vi "setSerializedData.vi"(0 "reference":refnum<class "ClassRelationshipEdge.lvclass">, 1 "startNode":refnum<class "AbstractNode.lvclass">, 2 "endNode":refnum<class "AbstractNode.lvclass">, 3 "xmlOut":string, 5 "error in (no error)":errorcluster) -> (14 "reference out":refnum<class "ClassRelationshipEdge.lvclass">, 19 "error out":errorcluster)   [LabVIEW 2020, in "ClassRelationshipEdge.lvclass"]
uses:
  <resource>/Framework/Providers/Open_GDS/UML/ClassRelationshipEdge_class/ClassRelationshipEdge.lvclass
  C:/Program Files (x86)/National Instruments/LabVIEW 2020/resource/Framework/Providers/Open_GDS/UML/SegmentedLineEdge_class/SegmentedLineEdge.lvclass
  C:/Program Files (x86)/National Instruments/LabVIEW 2020/resource/Framework/Providers/Open_GDS/UML/AbstractEdge_class/AbstractEdge.lvclass
  <resource>/Framework/Providers/Open_GDS/UML/AbstractNode_class/AbstractNode.lvclass
  <resource>/Framework/Providers/Open_GDS/UML/General/Point/Point Point2D.ctl
  <resource>/Framework/Providers/Open_GDS/UML/LineStyle_class/LineStyleType.ctl
  <resource>/Framework/Providers/Open_GDS/UML/ArrowHead_class/ArrowHeadType.ctl
  <resource>/Framework/Providers/Open_GDS/UML/BentStyle_class/BentStyleType.ctl
  <resource>/Framework/Providers/Open_GDS/UML/LineStyle_class/LineStyle.lvclass
  <resource>/Framework/Providers/Open_GDS/UML/ArrowHead_class/ArrowHead.lvclass
  <resource>/Framework/Providers/Open_GDS/UML/BentStyle_class/BentStyle.lvclass
  <resource>/Framework/Providers/Open_GDS/UML/SegmentedLineEdge_class/SegmentedLineEdge.lvclass
  <resource>/Framework/Providers/Open_GDS/UML/AbstractEdge_class/AbstractEdge.lvclass
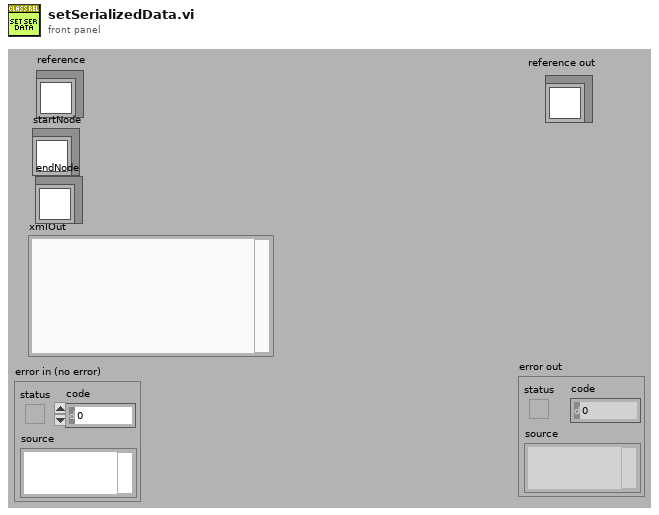
[diagram p1: front panel]
types:
  T1 = typedef "Point Point2D.ctl" = cluster{"x":dbl, "y":dbl}
  T2 = cluster{"Base class":cluster{"Base class":cluster{"Base class":cluster{"start":refnum<k1>, "end":refnum<k1>}}, "lineStyle":refnum<k1>, "startArrowHead":refnum<k1>, "endArrowHead":refnum<k1>, "startLabel":string, "midLabel":string, "endLabel":string, "MidLabelOffset":T1, "SplitWire":bool}, "bentStyleRef":refnum<k1>, "startConnectionOffset":cluster{"x":i32, "y":i32}, "endConnectionOffset":cluster{"x":i32, "y":i32}, "MidLineOffset":cluster{"x":i32, "y":i32}, "DepClass":cluster{"ThisVIs/Ctls":path[], "Dependent_VIs/Ctls":path[]}}
  T3 = typedef "ArrowHead.lvclass/ArrowHeadType.ctl" = enum16{"NONE", "TRIANGLE", "BLACK_TRIANGLE", "V", "HALF_V", "DIAMOND", "BLACK_DIAMOND"}
  T4 = typedef "BentStyle.lvclass/BentStyleType.ctl" = enum16{"STRAIGHT", "HV", "VH", "HVH", "VHV", "ARC"}
  T5 = typedef "LineStyle.lvclass/LineStyleType.ctl" = enum16{"SOLID", "DOTTED"}
  T6 = cluster{"Attributes":cluster{"Base class":cluster{"Base class":cluster{"Base class":cluster{"start":refnum<k1>, "end":refnum<k1>}}, "lineStyle":refnum<k1>, "startArrowHead":refnum<k1>, "endArrowHead":refnum<k1>, "startLabel":string, "midLabel":string, "endLabel":string, "MidLabelOffset":T1, "SplitWire":bool}, "bentStyleRef":refnum<k1>, "startConnectionOffset":cluster{"x":i32, "y":i32}, "endConnectionOffset":cluster{"x":i32, "y":i32}, "MidLineOffset":cluster{"x":i32, "y":i32}, "DepClass":cluster{"ThisVIs/Ctls":path[], "Dependent_VIs/Ctls":path[]}}, string, string, string, string}
  T7 = typedef "ClassRelationshipEdge.lvclass/ObjectAttributes.ctl" = cluster{"bentStyleRef":refnum<class "BentStyle.lvclass">, "startConnectionOffset":cluster{"x":i32, "y":i32}, "endConnectionOffset":cluster{"x":i32, "y":i32}, "MidLineOffset":cluster{"x":i32, "y":i32}, "DepClass":T8}
  T8 = typedef "ReversedEngineering_ViDependencyDetailsType.ctl" = cluster{"ThisVIs/Ctls":path[], "Dependent_VIs/Ctls":path[]}
  T9 = typedef "SegmentedLineEdge.lvclass/ObjectAttributes.ctl" = cluster{"lineStyle":refnum<class "LineStyle.lvclass">, "startArrowHead":refnum<class "ArrowHead.lvclass">, "endArrowHead":refnum<class "ArrowHead.lvclass">, "startLabel":string, "midLabel":string, "endLabel":string, "MidLabelOffset":T1, "SplitWire":bool}
  T10 = typedef "AbstractEdge.lvclass/ObjectAttributes.ctl" = cluster{"start":refnum<class "AbstractNode.lvclass">, "end":refnum<class "AbstractNode.lvclass">}
  T11 = cluster{"ThisVIs/Ctls":path[], "Dependent_VIs/Ctls":path[]}
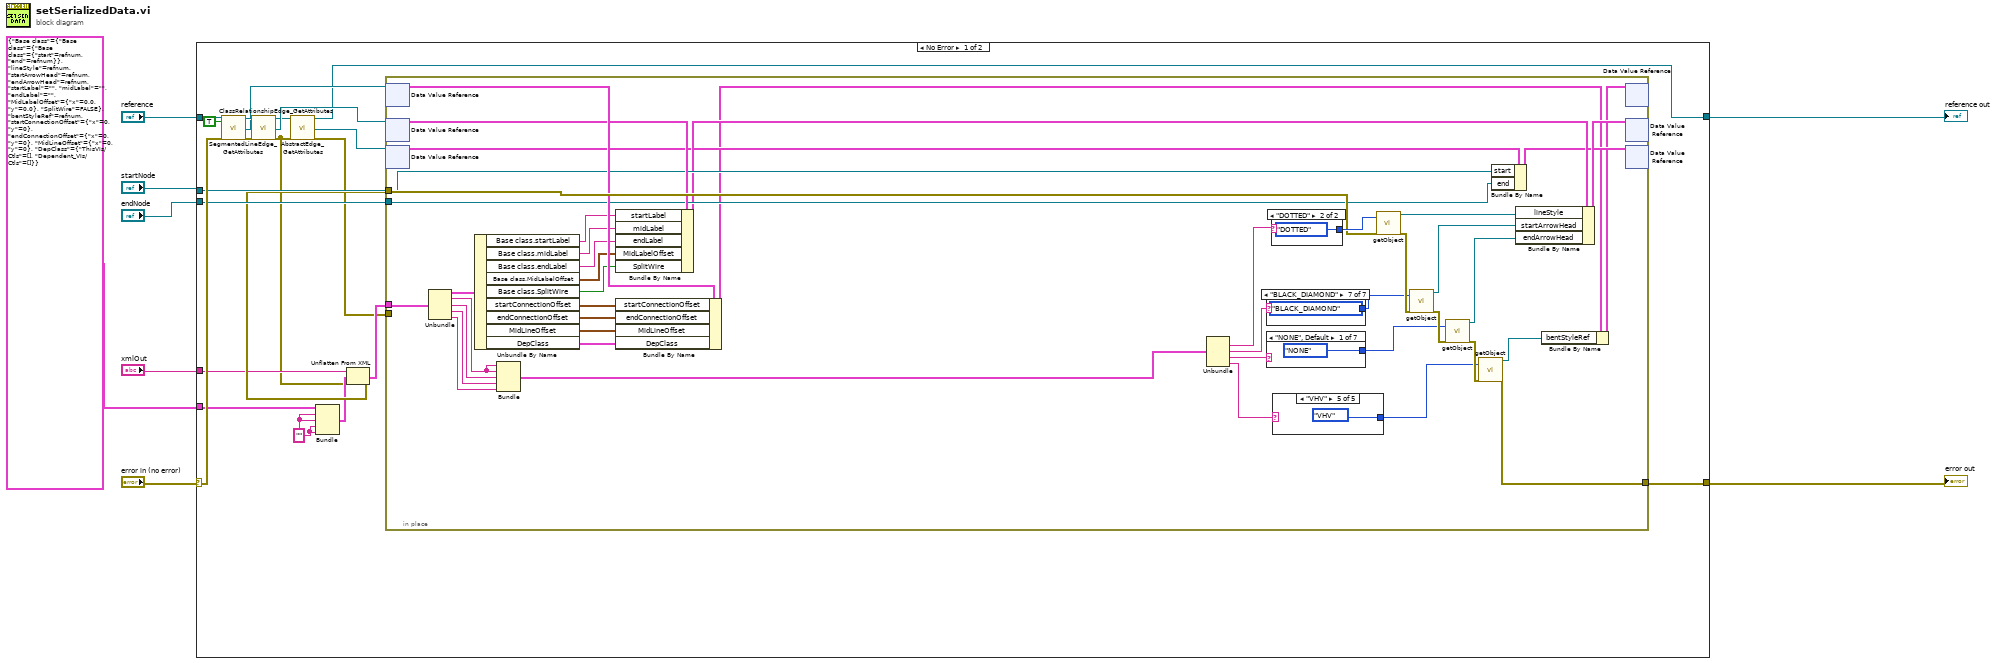
[diagram p0: block diagram]
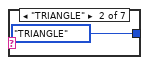
[diagram p2: hidden frame]
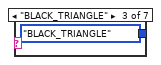
[diagram p3: hidden frame]
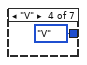
[diagram p4: hidden frame]
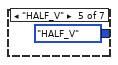
[diagram p5: hidden frame]
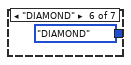
[diagram p6: hidden frame]
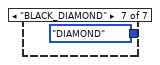
[diagram p7: hidden frame]
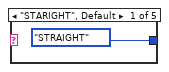
[diagram p8: hidden frame]
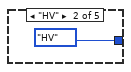
[diagram p9: hidden frame]
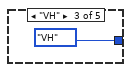
[diagram p10: hidden frame]
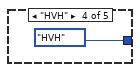
[diagram p11: hidden frame]
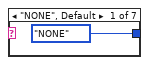
[diagram p12: hidden frame]
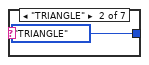
[diagram p13: hidden frame]
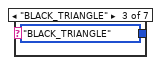
[diagram p14: hidden frame]
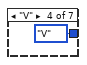
[diagram p15: hidden frame]
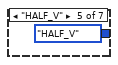
[diagram p16: hidden frame]
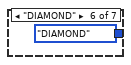
[diagram p17: hidden frame]
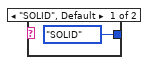
[diagram p18: hidden frame]
diagram:
  n1 = case shown="No Error" "error in (no error)" {
    selector: "error in (no error)" -> [w28 w94]
    tunnel: "reference" -> [w29 w95]
    tunnel: [w9 w95] -> w6
    tunnel: [w16 w94] -> w5
    tunnel: "xmlOut" -> [w18 _]
    tunnel: "startNode" -> [w27 _]
    tunnel: "endNode" -> [w26 _]
    tunnel: T2 {"Base class"={"Base class"={"Base class"={"start"=refnum, "end"=refnum}}, "lineStyle"=refnum, "startArrowHead"=refnum, "endArrowHead"=refnum, "startLabel"="", "midLabel"="", "endLabel"="", "MidLabelOffset"={"x"=0.0, "y"=0.0}, "SplitWire"=FALSE}, "bentStyleRef"=refnum, "startConnectionOffset"={"x"=0, "y"=0}, "endConnectionOffset"={"x"=0, "y"=0}, "MidLineOffset"={"x"=0, "y"=0}, "DepClass"={"ThisVIs/Ctls"=[], "Dependent_VIs/Ctls"=[]}} ("Attributes") -> [w24 _]
    frame No Error {
      w25 = ""
      n2 = call <resource>:"ClassRelationshipEdge_GetAttributes.vi"("reference in"=w29, "OnlyGetDvrReference(False)"=TRUE, "error in (no error)"=w28) -> ("reference out"=w22:refnum<class "ClassRelationshipEdge.lvclass">, "DataRef"=w13:refnum<data-value>, "error out"=w21:errorcluster)  [unwired: 13 in, 1 out]
      n3 = call <resource>:"SegmentedLineEdge_GetAttributes.vi"("reference in"=w22, "error in (no error)"=w21) -> ("reference out"=w10:refnum<class "ClassRelationshipEdge.lvclass">, "DataRef"=w12:refnum<data-value>, "error out"=w15:errorcluster)  [unwired: 14 in, 1 out]
      n4 = call <resource>:"AbstractEdge_GetAttributes.vi"("reference in"=w10, "error in (no error)"=w15) -> ("reference out"=w9:refnum<class "ClassRelationshipEdge.lvclass">, "DataRef"=w11:refnum<data-value>, "error out"=w14:errorcluster)  [unwired: 14 in, 1 out]
      n5 = Bundle("Attributes"=w24, w25, w25, w25, w25) -> (w17:T6)  [unwired: 1 out]
      n6 = Unflatten From XML(xml string=w18, type=w17, error in (no error)=w15) -> (value=w19:T6, error out=w20:errorcluster)
      n7 = in-place {
        in-place-border: w27 -> [w53]
        in-place-border: w26 -> [w52]
        in-place-border: w20 -> [w57]
        in-place-border: w19 -> [w58]
        in-place-border: w14 -> [_]
        in-place-border: [w56] -> w16
        n8 = in-place-dvr #1(w13) -> (w55:T7)  [unwired: 1 out]
        n9 = in-place-dvr #2(w12) -> (w54:T9)  [unwired: 1 out]
        n10 = in-place-dvr #3(w11) -> (w49:T10)  [unwired: 1 out]
        n11 = Unbundle(w58) -> ("Attributes"=w41:T2, w31:string, w42:string, w43:string, w44:string)
        n12 = Unbundle By Name(w41) -> ("Base class.startLabel"=w40:string, "Base class.midLabel"=w39:string, "Base class.endLabel"=w38:string, "Base class.MidLabelOffset"=w37:T1, "Base class.SplitWire"=w36:bool, "startConnectionOffset"=w35:cluster{"x":i32, "y":i32}, "endConnectionOffset"=w34:cluster{"x":i32, "y":i32}, "MidLineOffset"=w33:cluster{"x":i32, "y":i32}, "DepClass"=w32:T11)
        n13 = Bundle(w31, w31, w42, w43, w44) -> (w30:cluster{string, string, string, string, string})  [unwired: 1 out]
        n14 = Bundle By Name(cluster=w54, "startLabel"=w40, "midLabel"=w39, "endLabel"=w38, "MidLabelOffset"=w37, "SplitWire"=w36) -> (w50:T9)
        n15 = Bundle By Name(cluster=w55, "startConnectionOffset"=w35, "endConnectionOffset"=w34, "MidLineOffset"=w33, "DepClass"=w32) -> (w46:T7)
        n16 = Unbundle(w30) -> (w66:string, w62:string, w60:string, w61:string)  [unwired: 1 out]
        n17 = case shown="\"BLACK_DIAMOND\"" w62 {
          tunnel: [ArrowHeadType."NONE" ("arrowHead") ArrowHeadType."TRIANGLE" ("arrowHead") ArrowHeadType."BLACK_TRIANGLE" ("arrowHead") ArrowHeadType."V" ("arrowHead") ArrowHeadType."HALF_V" ("arrowHead") ArrowHeadType."DIAMOND" ("arrowHead") ArrowHeadType."BLACK_DIAMOND" ("arrowHead")] -> w64
          frame "NONE", Default {
          }
          frame "TRIANGLE" {
          }
          frame "BLACK_TRIANGLE" {
          }
          frame "V" {
          }
          frame "HALF_V" {
          }
          frame "DIAMOND" {
          }
          frame "BLACK_DIAMOND" {
          }
        }
        n18 = case shown="\"NONE\", Default" w60 {
          tunnel: [ArrowHeadType."NONE" ("arrowHead") ArrowHeadType."TRIANGLE" ("arrowHead") ArrowHeadType."BLACK_TRIANGLE" ("arrowHead") ArrowHeadType."V" ("arrowHead") ArrowHeadType."HALF_V" ("arrowHead") ArrowHeadType."DIAMOND" ("arrowHead") ArrowHeadType."DIAMOND" ("arrowHead")] -> w59
          frame "NONE", Default {
          }
          frame "TRIANGLE" {
          }
          frame "BLACK_TRIANGLE" {
          }
          frame "V" {
          }
          frame "HALF_V" {
          }
          frame "DIAMOND" {
          }
          frame "BLACK_DIAMOND" {
          }
        }
        n19 = case shown="\"DOTTED\"" w66 {
          tunnel: [LineStyleType."SOLID" ("lineStyle") LineStyleType."DOTTED" ("lineStyle")] -> w65
          frame "SOLID", Default {
          }
          frame "DOTTED" {
          }
        }
        n20 = case shown="\"VHV\"" w61 {
          tunnel: [BentStyleType."STRAIGHT" ("bentStyle") BentStyleType."HV" ("bentStyle") BentStyleType."VH" ("bentStyle") BentStyleType."HVH" ("bentStyle") BentStyleType."VHV" ("bentStyle")] -> w63
          frame "STARIGHT", Default {
          }
          frame "HV" {
          }
          frame "VH" {
          }
          frame "HVH" {
          }
          frame "VHV" {
          }
        }
        n21 = call <resource>:"getObject.vi"("lineStyle"=w65, "error in (no error)"=w57) -> ("reference out"=w72:refnum<class "LineStyle.lvclass">, "error out"=w71:errorcluster)  [unwired: 16 out]
        n22 = call <resource>:"getObject.vi"("arrowHead"=w64, "error in (no error)"=w71) -> ("reference out"=w68:refnum<class "ArrowHead.lvclass">, "error out"=w70:errorcluster)  [unwired: 16 out]
        n23 = call <resource>:"getObject.vi"("arrowHead"=w59, "error in (no error)"=w70) -> ("reference out"=w69:refnum<class "ArrowHead.lvclass">, "error out"=w67:errorcluster)  [unwired: 16 out]
        n24 = call <resource>:"getObject.vi"("bentStyle"=w63, "error in (no error)"=w67) -> ("reference out"=w45:refnum<class "BentStyle.lvclass">, "error out"=w56:errorcluster)  [unwired: 16 out]
        n25 = Bundle By Name(cluster=w49, "start"=w53, "end"=w52) -> (w48:T10)
        n26 = Bundle By Name(cluster=w50, "lineStyle"=w72, "startArrowHead"=w68, "endArrowHead"=w69) -> (w51:T9)
        n27 = Bundle By Name(cluster=w46, "bentStyleRef"=w45) -> (w47:T7)
        n28 = in-place-dvr #1(w47) -> ()  [unwired: 2 out]
        n29 = in-place-dvr #2(w51) -> ()  [unwired: 2 out]
        n30 = in-place-dvr #3(w48) -> ()  [unwired: 2 out]
      }
    }
    frame Error {
    }
  }
  "reference out" <- w6
  "error out" <- w5
